vi "number5-sub1.vi"(3 "Numeric":i32, 4 "Numeric 2":i32, 6 "array":i32[][](array[numeric])) -> (1 "index of element":i32)   [LabVIEW 2014]
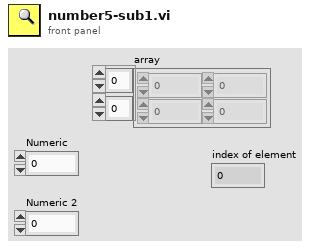
[diagram p1: front panel]
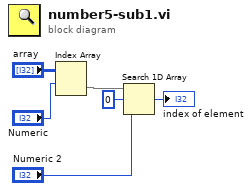
[diagram p0: block diagram]
diagram:
  n1 = Index Array(array="array", index (row)="Numeric") -> (element=w4:i32[])  [unwired: 1 in]
  n2 = Search 1D Array(1D array=w4, element=0, start index (0)="Numeric 2") -> (index of element=→"index of element":i32)
